vi "Prep HW Components.vi"() -> (0 "error out":errorcluster, 3 "Recipe Comps":T1)   [LabVIEW 2022 SP3]
uses:
  Recipe Comps.ctl
  Laser/Laser View/Laser View.lvclass
  Laser/Laser Controller/Laser Controller.lvclass
  C:/XY Stage/Laser/Laser Controller api/Laser API.lvclass
  Camera/Camera Controller/Camera Controller.lvclass
  Camera/Camera View/Camera View.lvclass
  IO Monitor/DAQ Controller/DAQ Controller.lvclass
  C:/XY Stage/IO Monitor/DAQ API/DAQ API.lvclass
  IO Monitor/Class 3/DAQ View.lvclass
  XY Stage/Process Actor/View/XY Stage Class/XY Stage Class.lvclass
  XY Stage/Process Actor/XY Controller/XY Stage Controller/XY Stage Controller.lvclass
  XY Stage/Axis Objects/Axis Factory/Axis Factory.lvclass
  Camera/Driver Factories/abstract camera factory/abstract camera driver factory.lvclass
  Laser/abstract laser driver factory/abstract laser driver factory.lvclass
  IO Monitor/abstract IO Factory/abstract IO Factory.lvclass
  a92721d6-27c2-496b-abd3-c8dd0bd5b1ec.vi
  dff9869b-1d19-409b-ba6c-92a42f9f1f15.vi
  80d0b246-6eac-459c-9644-077db03a302d.vi
  5872a8ad-3df5-47aa-add9-d565f396eee0.vi
  10803332-7268-4fd9-a5ce-e9a0206a4d14.vi
  <vilib>/Utility/LVClass/Get LV Class Default Value.vi
  Camera/Camera View/Accessors/Write Camera Controller.lvclass.vi
  XY Stage/Framework/Read Configs/Read Configs Sections.lvlib
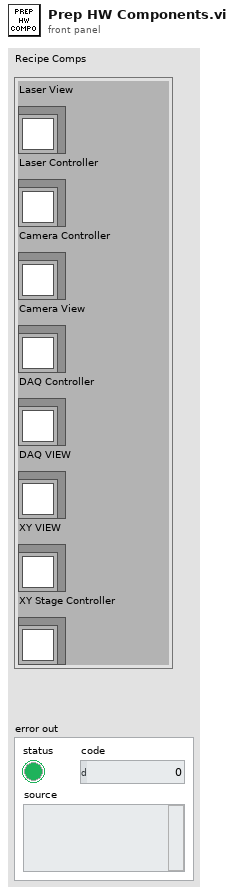
[diagram p1: front panel]
types:
  T1 = typedef "Recipe Comps.ctl" = cluster{"Laser View":refnum<class "Laser View.lvclass">, "Laser Controller ":refnum<class "Laser Controller.lvclass">, "Camera Controller":refnum<class "Camera Controller.lvclass">, "Camera View":refnum<class "Camera View.lvclass">, "DAQ Controller":refnum<class "DAQ Controller.lvclass">, "DAQ VIEW":refnum<class "DAQ View.lvclass">, "XY VIEW":refnum<class "XY Stage Class.lvclass">, "XY Stage Controller":refnum<class "XY Stage Controller.lvclass">}
  T2 = typedef "Read Configs Sections.lvlib/Section Data.ctl" = cluster{"Path":path, "Section":string}
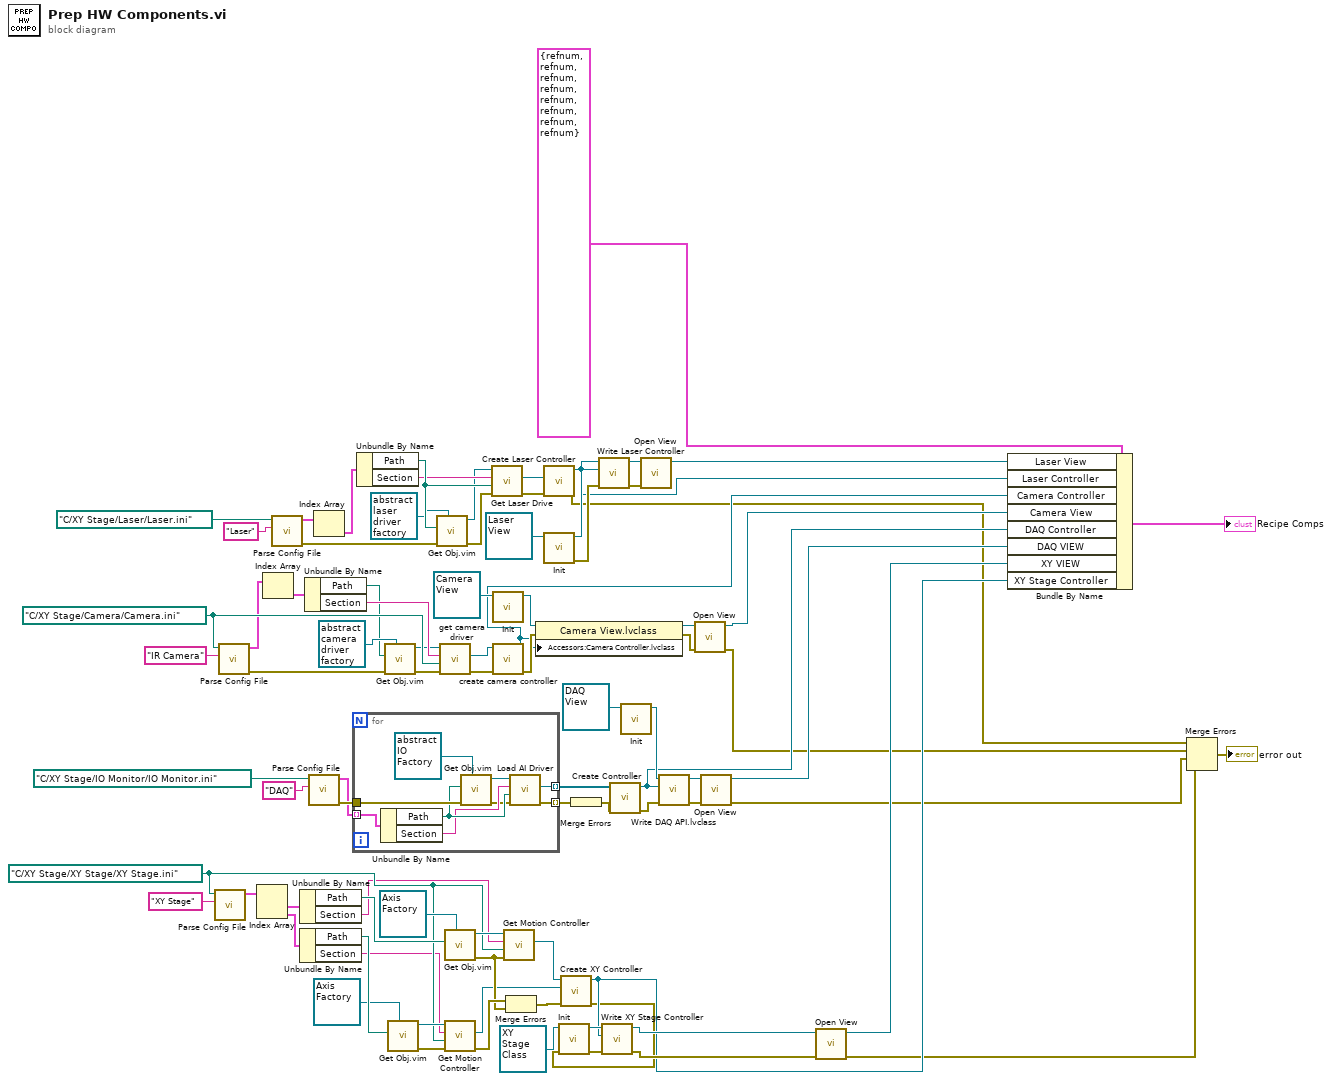
[diagram p0: block diagram]
diagram:
  w48 = path "C:/XY Stage/Camera/Camera.ini" ("Config Path")
  w26 = path "C:/XY Stage/XY Stage/XY Stage.ini" ("Config Path")
  # "S"
  n1 = call "Parse Config File.vi"("Section"="XY Stage", "Config Path"=w26) -> ("Array"=w17:T2[])  [unwired: 8 in, 1 out]
  n2 = call "Parse Config File.vi"("Section"="IR Camera", "Config Path"=w48) -> ("error out"=w49:errorcluster, "Array"=w41:T2[])  [unwired: 8 in]
  n3 = Index Array(array=w17) -> (element #1=w18:T2, element #2=w19:T2)  [unwired: 2 in]
  n4 = Index Array(array=w41) -> (element=w42:T2)  [unwired: 1 in]
  n5 = call "Parse Config File.vi"("Section"="Laser", "Config Path"=path "C:/XY Stage/Laser/Laser.ini") -> ("error out"=w62:errorcluster, "Array"=w58:T2[])  [unwired: 8 in]
  n6 = Unbundle By Name(w18) -> ("Path"=w28:path, "Section"=w23:string)
  n7 = Unbundle By Name(w19) -> ("Path"=w32:path, "Section"=w24:string)
  n8 = Unbundle By Name(w42) -> ("Path"=w44:path, "Section"=w47:string)
  n9 = call "Parse Config File.vi"("Section"="DAQ", "Config Path"=path "C:/XY Stage/IO Monitor/IO Monitor.ini") -> ("error out"=w78:errorcluster, "Array"=w75:T2[])  [unwired: 8 in]
  n10 = Index Array(array=w58) -> (element=w59:T2)  [unwired: 1 in]
  n11 = for {
    tunnel: w75 -> [w95] mode=indexing
    tunnel: w78 -> [w94]
    tunnel: [w89] -> w79 mode=indexing
    tunnel: [w87] -> w84 mode=indexing
    n12 = Unbundle By Name(w95) -> ("Path"=w91:path, "Section"=w90:string)
    n13 = call "Get Obj.vim"("LabVIEW Object 2"=refnum<class "abstract IO Factory.lvclass"> refnum ("abstract IO Factory.lvclass"), "error in (no error)"=w94, "Path"=w91) -> ("error out"=w88:errorcluster, "LabVIEW Object"=w92:refnum<class "abstract IO Factory.lvclass">)  [unwired: 7 in]
    n14 = call-dynamic "Load AI Driver.vi"("error in (no error)"=w88, "Config Path"=w91, "Section"=w90, "abstract IO Factory in"=w92) -> ("error out"=w87:errorcluster, "AI Driver.lvclass"=w89:refnum<class "AI Driver.lvclass">)  [unwired: 6 in]
  }
  n15 = Unbundle By Name(w59) -> ("Path"=w67:path, "Section"=w66:string)
  n16 = call "Get Obj.vim"("LabVIEW Object 2"=refnum<class "abstract camera driver factory.lvclass"> refnum ("abstract camera driver factory.lvclass"), "error in (no error)"=w49, "Path"=w44) -> ("error out"=w50:errorcluster, "LabVIEW Object"=w46:refnum<class "abstract camera driver factory.lvclass">)  [unwired: 7 in]
  n17 = call "Get Obj.vim"("LabVIEW Object 2"=refnum<class "Axis Factory.lvclass"> refnum ("Axis Factory.lvclass"), "Path"=w32) -> ("error out"=w34:errorcluster, "LabVIEW Object"=w33:refnum<class "Axis Factory.lvclass">)  [unwired: 8 in]
  n18 = call "Get Obj.vim"("LabVIEW Object 2"=refnum<class "abstract laser driver factory.lvclass"> refnum ("abstract laser driver factory.lvclass"), "error in (no error)"=w62, "Path"=w67) -> ("error out"=w65:errorcluster, "LabVIEW Object"=w64:refnum<class "abstract laser driver factory.lvclass">)  [unwired: 7 in]
  n19 = call-dynamic "get camera driver.vi"("error in (no error)"=w50, "Path"=w48, "Section"=w47, "abstract camera driver factory in"=w46) -> ("error out"=w52:errorcluster, "Camera Driver.lvclass"=w51:refnum<class "Camera Driver.lvclass">)  [unwired: 6 in]
  n20 = call "Get Obj.vim"("LabVIEW Object 2"=refnum<class "Axis Factory.lvclass"> refnum ("Axis Factory.lvclass"), "Path"=w28) -> ("error out"=w30:errorcluster, "LabVIEW Object"=w29:refnum<class "Axis Factory.lvclass">)  [unwired: 8 in]
  n21 = call-dynamic "Get Motion Controller.vi"("error in (no error)"=w34, "Path"=w26, "Section"=w24, "Axis Factory in"=w33) -> ("error out"=w35:errorcluster, "iMotion Controller.lvclass"=w25:refnum<class "iMotion Controller.lvclass">)  [unwired: 5 in, 1 out]
  n22 = call-dynamic "Get Laser Drive.vi"("error in (no error)"=w65, "Path"=w67, "Section"=w66, "abstract laser driver factory in"=w64) -> ("error out"=w69:errorcluster, "Laser Driver.lvclass"=w68:refnum<class "Laser Driver.lvclass">)  [unwired: 6 in]
  n23 = call-dynamic "Init.vi"("Camera View in"=refnum<class "Camera View.lvclass"> refnum ("Camera View.lvclass")) -> ("Camera View out"=w54:refnum<class "Camera View.lvclass">)  [unwired: 9 in, 1 out]
  n24 = call "create camera controller.vi"("error in (no error)"=w52, "Camera Driver.lvclass"=w51) -> ("error out"=w56:errorcluster, "Camera Controller out"=w12:refnum<class "Camera Controller.lvclass">)  [unwired: 8 in]
  n25 = call-dynamic "Get Motion Controller.vi"("error in (no error)"=w30, "Path"=w26, "Section"=w23, "Axis Factory in"=w29) -> ("iMotion Controller.lvclass"=w22:refnum<class "iMotion Controller.lvclass">)  [unwired: 5 in, 2 out]
  n26 = Merge Errors(w35, w30) -> (w21:errorcluster)
  n27 = property class="Camera View.lvclass"(reference=w54, error in=w56, "Accessors:Camera Controller.lvclass"=w12) -> (reference out=w55:refnum<class "Camera View.lvclass">, error out=w57:errorcluster)
  n28 = call "Create Laser Controller.vi"("error in (no error)"=w69, "Laser Driver.lvclass"=w68) -> ("error out"=w6:errorcluster, "Laser Controller out"=w13:refnum<class "Laser Controller.lvclass">)  [unwired: 8 in]
  n29 = call-dynamic "Init.vi"("Laser View in"=refnum<class "Laser View.lvclass"> refnum ("Laser View.lvclass")) -> ("error out"=w73:errorcluster, "Laser View out"=w71:refnum<class "Laser View.lvclass">)  [unwired: 9 in]
  n30 = call "Create XY Controller.vi"("error in (no error)"=w21, "Y-Axis"=w25, "X-Axis"=w22) -> ("error out"=w3:errorcluster, "XY Stage Controller out"=w8:refnum<class "XY Stage Controller.lvclass">)  [unwired: 7 in]
  n31 = call-dynamic "Init.vi"("error in (no error)"=w3, "XY Stage Class in"=refnum<class "XY Stage Class.lvclass"> refnum ("XY Stage Class.lvclass")) -> ("error out"=w40:errorcluster, "XY Stage Class out"=w37:refnum<class "XY Stage Class.lvclass">)  [unwired: 8 in]
  n32 = Merge Errors(w84) -> (w83:errorcluster)
  n33 = call "Write Laser Controller.vi"("error in (no error)"=w73, "Laser API.lvclass"=w13, "In"=w71) -> ("error out"=w74:errorcluster, "Out"=w72:refnum<class "Laser View.lvclass">)  [unwired: 7 in]
  n34 = call "Write XY Stage Controller.vi"("error in (no error)"=w40, "XY Stage Controller"=w8, "In"=w37) -> ("error out"=w39:errorcluster, "Out"=w38:refnum<class "XY Stage Class.lvclass">)  [unwired: 7 in]
  n35 = call "Create Controller.vi"("error in (no error)"=w83, "AI Driver"=w79) -> ("error out"=w85:errorcluster, "DAQ Controller out"=w10:refnum<class "DAQ Controller.lvclass">)  [unwired: 8 in]
  n36 = call-dynamic "Init.vi"("DAQ View in"=refnum<class "DAQ View.lvclass"> refnum) -> ("DAQ View out"=w81:refnum<class "DAQ View.lvclass">)  [unwired: 9 in, 1 out]
  n37 = call-dynamic "Open View.vi"("error in (no error)"=w74, "base view in"=w72) -> ("base view out"=w14:refnum<class "Laser View.lvclass">)  [unwired: 8 in, 1 out]
  n38 = call "Write DAQ API.lvclass.vi"("error in (no error)"=w85, "DAQ API.lvclass"=w10, "In"=w81) -> ("error out"=w86:errorcluster, "Out"=w82:refnum<class "DAQ View.lvclass">)  [unwired: 7 in]
  n39 = call-dynamic "Open View.vi"("error in (no error)"=w57, "base view in"=w55) -> ("error out"=w5:errorcluster, "base view out"=w11:refnum<class "Camera View.lvclass">)  [unwired: 8 in]
  n40 = call-dynamic "Open View.vi"("error in (no error)"=w86, "base view in"=w82) -> ("error out"=w4:errorcluster, "base view out"=w7:refnum<class "DAQ View.lvclass">)  [unwired: 8 in]
  n41 = call-dynamic "Open View.vi"("error in (no error)"=w39, "base view in"=w38) -> ("error out"=w2:errorcluster, "base view out"=w9:refnum<class "XY Stage Class.lvclass">)  [unwired: 8 in]
  n42 = Bundle By Name(cluster=T1 {"Laser View"=refnum, "Laser Controller "=refnum, "Camera Controller"=refnum, "Camera View"=refnum, "DAQ Controller"=refnum, "DAQ VIEW"=refnum, "XY VIEW"=refnum, "XY Stage Controller"=refnum} ("Cluster"), "Laser View"=w14, "Laser Controller"=w13, "Camera Controller"=w12, "Camera View"=w11, "DAQ Controller"=w10, "DAQ VIEW"=w7, "XY VIEW"=w9, "XY Stage Controller"=w8) -> (→"Recipe Comps":T1)
  n43 = Merge Errors(w6, w5, w4, w2) -> (→"error out":errorcluster)
